vi "Bounds.vi"(1 "XRef":refnum<vi>, 2 "State In":T2) -> (0 "Bounds":cluster{"Width":T1, "Height":T1})   [LabVIEW 2015, in "Async-And-Forget.xnode"]
doc: "This ability VI is used to tell LabVIEW your current bounds. If you want to update your bounds, you must inform LabVIEW through the UpdateImageAndBounds reply of another ability VI. If you change your bounds, you will also probably want to update your image.\n\nDefault behavior: None.\n\nThis ability does not provide UI and OS messages are not handled."
uses:
  Async-And-Forget.xnode
  State.ctl
  <vilib>/Utility/miscctls.llb/LVRectTypeDef.ctl
  <vilib>/picture/picture.llb/imagedata.ctl
  <vilib>/XNodeSupport/XNodeInt.ctl
  <vilib>/XNodeSupport/NI_XNodeSupport.lvlib
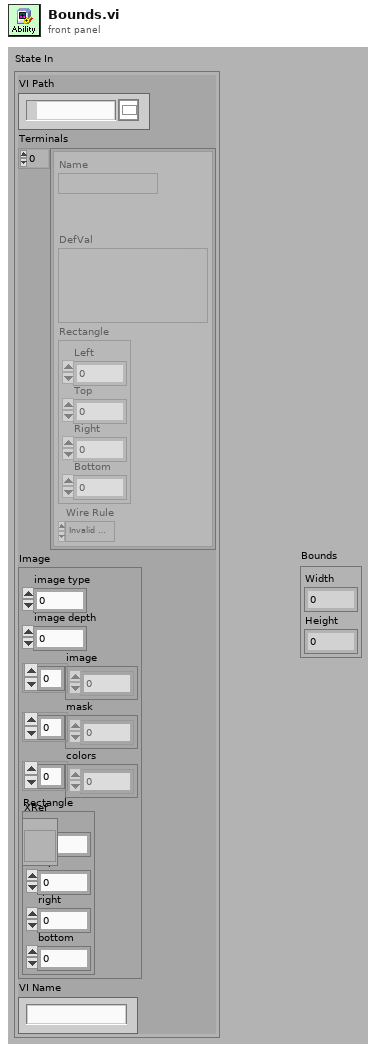
[diagram p1: front panel]
types:
  T1 = typedef "NI_XNodeSupport.lvlib/XNodeInt.ctl" = i32
  T2 = typedef "Async-And-Forget.xnode/State.ctl" = cluster{"VI Path":path, "Terminals":cluster{"Name":string, "DefVal":variant, "Rectangle":T3, "Wire Rule":enum16{"Invalid Wire Rule", "Required", "Recommended", "Optional", "Dynamic Dispatch"}}[], "Image":T4, "VI Name":string}
  T3 = typedef "LVRectTypeDef.ctl" = cluster{"Left":i16, "Top":i16, "Right":i16, "Bottom":i16}
  T4 = typedef "imagedata.ctl" = cluster{"image type":i32, "image depth":i32, "image":u8[], "mask":u8[], "colors":u32[], "Rectangle":cluster{"left":i16, "top":i16, "right":i16, "bottom":i16}}
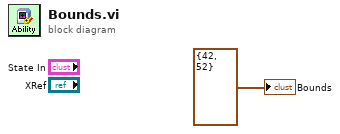
[diagram p0: block diagram]
diagram:
  "Bounds" <- cluster{"Width":T1, "Height":T1} {"Width"=42, "Height"=52} ("Bounds")
